vi "Modbus_spy_new.vi"() -> ()   [LabVIEW 2012]
uses:
  Controls/MBA_data.ctl
  <vilib>/Instr/_visa.llb/VISA Configure Serial Port (Instr).vi
panel:
  in  "string":string
  out "MBA data":T1
  in  "Стоп":bool
  out "substring":string
  out "error out":errorcluster
  in  "error in (no error)":errorcluster
  in  "flow control":u16(ring) items=["None"=0, "XON/XOFF"=1, "RTS/CTS"=2, "DTR/DSR"=4]
  in  "stop bits":u16(ring)=20 items=["1.0"=10, "1.5"=15, "2.0"=20]
  in  "parity":u16(ring) items=["None", "Odd", "Even", "Mark", "Space"]
  in  "data bits":u16=8 min=5 max=8 step=1
  in  "VISA resource name":refnum<visa-resource-name>="COM2"
  in  "baud rate":u32=19200
  # "ch1 Т 80л\nch2 нет\nch3 Вытяжка\nch4 Т 30л\nch5 Т 800л\nch6 Охлаждение\nch7 Барботаж\nch8 Т 2000л"
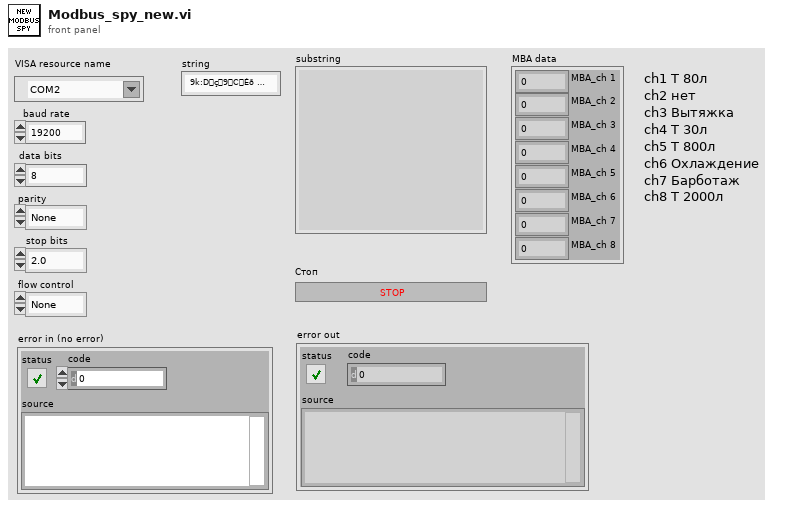
[diagram p1: front panel]
types:
  T1 = typedef "MBA_data.ctl" = cluster{"MBA_ch 1":dbl, "MBA_ch 2":dbl, "MBA_ch 3":dbl, "MBA_ch 4":dbl, "MBA_ch 5":dbl, "MBA_ch 6":dbl, "MBA_ch 7":dbl, "MBA_ch 8":dbl}
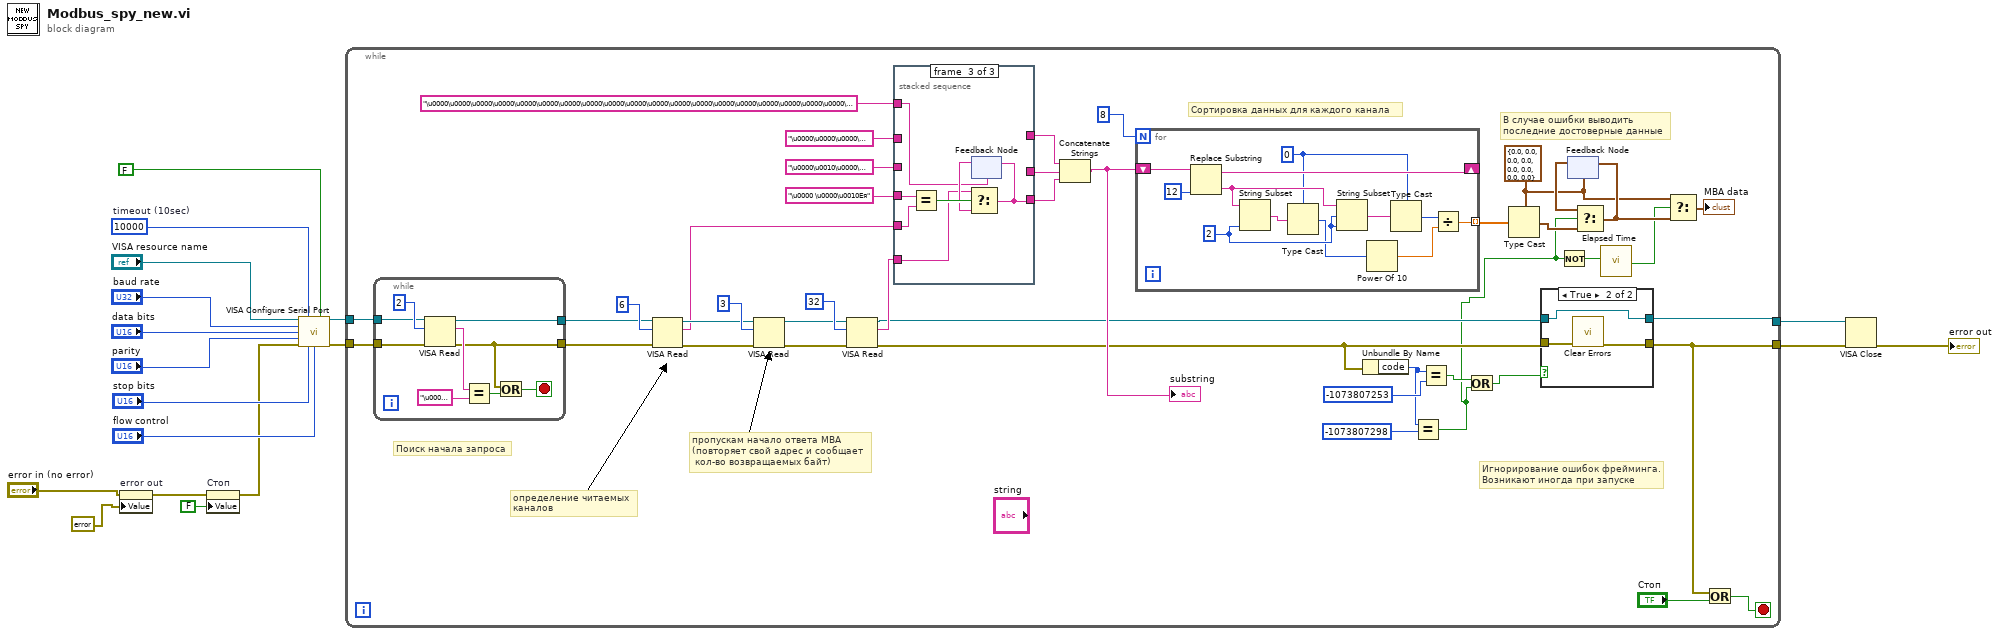
[diagram p0: block diagram]
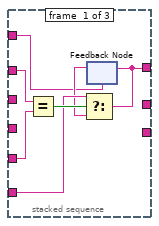
[diagram p3: hidden frame]
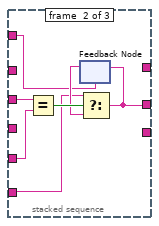
[diagram p4: hidden frame]
diagram:
  w15 = u32 10000  # timeout (10sec)
  n1 = property on="error out" class="Clust (strict)"(error in="error in (no error)", "Value"=errorcluster {"status"=FALSE, "code"=0, "source"=""} ("error in (no error)")) -> (error out=w2:errorcluster)  [unwired: 1 in, 1 out]
  n2 = property on="Стоп" class="Bool (strict)"(error in=w2, "Value"=FALSE ("Стоп")) -> (error out=w5:errorcluster)  [unwired: 1 in, 1 out]
  n3 = call-poly "VISA Configure Serial Port"("VISA resource name"="VISA resource name", "timeout (10sec)"=w15, "Enable Termination\nChar (T)"=FALSE ("Enable Termination\nChar (T)"), "baud rate (9600)"="baud rate", "data bits (8)"="data bits", "parity (0:none)"="parity", "error in (no error)"=w5, "stop bits (10: 1 bit)"="stop bits", "flow control (0:none)"="flow control") -> ("VISA resource name out"=w9:refnum<visa-resource-name>, "error out"=w10:errorcluster)  [unwired: 5 out]
  n4 = while {
    tunnel: w10 -> [w38]
    tunnel: w9 -> [w37]
    tunnel: [w30] -> w8
    tunnel: [w34] -> w7
    stop <- w31 stop-if-true
    w22 = T1 {"MBA_ch 1"=0.0, "MBA_ch 2"=0.0, "MBA_ch 3"=0.0, "MBA_ch 4"=0.0, "MBA_ch 5"=0.0, "MBA_ch 6"=0.0, "MBA_ch 7"=0.0, "MBA_ch 8"=0.0} ("MBA data")
    # "Игнорирование ошибок фрейминга.\nВозникают иногда при запуске"
    # "В случае ошибки выводить \nпоследние достоверные данные"
    # "Сортировка данных для каждого канала"
    # "пропускам начало ответа МВА\n(повторяет свой адрес и сообщает\n кол-во возвращаемых байт)"
    # "определение читаемых \nканалов"
    # "Поиск начала запроса"
    n5 = while {
      tunnel: [w106] -> w59
      tunnel: [w101] -> w58
      tunnel: w38 -> [w100]
      tunnel: w37 -> [w99]
      stop <- w103 stop-if-true
      n6 = VISA Read(VISA resource name=w99, byte count=u32 2, error in (no error)=w100) -> (VISA resource name out=w106:refnum<visa-resource-name>, read buffer=w104:string, error out=w101:errorcluster)  [unwired: 1 out]
      n7 = Equal?(x=w104, y="\u0002\u0003" ("string")) -> (x = y?=w102:bool)
      n8 = Or(x=w101, y=w102) -> (x .or. y?=w103:bool)
    }
    n9 = VISA Read(VISA resource name=w59, byte count=u32 6, error in (no error)=w58) -> (VISA resource name out=w56:refnum<visa-resource-name>, read buffer=w54:string, error out=w55:errorcluster)  [unwired: 1 out]
    n10 = VISA Read(VISA resource name=w56, byte count=u32 3, error in (no error)=w55) -> (VISA resource name out=w51:refnum<visa-resource-name>, error out=w52:errorcluster)  [unwired: 2 out]
    n11 = VISA Read(VISA resource name=w51, byte count=u32 32, error in (no error)=w52) -> (VISA resource name out=w35:refnum<visa-resource-name>, read buffer=w50:string, error out=w33:errorcluster)  [unwired: 1 out]
    n12 = stacked-sequence {
      tunnel: w54 -> [w84 w88 w95]
      tunnel: w50 -> [w81 w89 w96]
      tunnel: "\u0000\u0000\u0000\u0010D5" ("string") -> [w83 _ _]
      tunnel: "\u0000\u0010\u0000\u0010Eр" ("string") -> [_ w87 _]
      tunnel: "\u0000 \u0000\u0010Eя" ("string") -> [_ _ w94]
      tunnel: [w79 _ _] -> w44
      tunnel: [_ w86 _] -> w46
      tunnel: [_ _ w93] -> w45
      tunnel: "\u0000\u0000\u0000\u0000\u0000\u0000\u0000\u0000\u0000\u0000\u0000\u0000\u0000\u0000\u0000\u0000\u0000\u0000\u0000\u0000\u0000\u0000\u0000\u0000\u0000\u0000\u0000\u0000\u0000\u0000\u0000\u0000" ("string") -> [w78 w85 w92]
      frame #0 {
        n13 = Equal?(x=w83, y=w84) -> (x = y?=w82:bool)
        n14 = feedback #1(w78) -> (w80:string)
        n15 = Select(t=w81, s=w82, f=w80) -> (s? t:f=w79:string)
        n16 = feedback-in #1(w79) -> ()
      }
      frame #1 {
        n17 = Equal?(x=w87, y=w88) -> (x = y?=w91:bool)
        n18 = feedback #2(w85) -> (w90:string)
        n19 = Select(t=w89, s=w91, f=w90) -> (s? t:f=w86:string)
        n20 = feedback-in #2(w86) -> ()
      }
      frame #2 {
        n21 = Equal?(x=w94, y=w95) -> (x = y?=w98:bool)
        n22 = feedback #3(w92) -> (w97:string)
        n23 = Select(t=w96, s=w98, f=w97) -> (s? t:f=w93:string)
        n24 = feedback-in #3(w93) -> ()
      }
    }
    n25 = Concatenate Strings(w44, w46, w45) -> (w39:string)
    "substring" <- w39
    n26 = for {
      N: 8 -> [_]
      shift-right: [w75] -> _
      shift-left: w39 -> [w77]
      tunnel: [w66] -> w42 mode=indexing
      w70 = i16 0
      w73 = 2 ("length (rest)")
      n27 = Replace Substring(2:12 ("length (len. of substring)"), 5:w77) -> (0:w72:string, 1:w75:string)  [unwired: 2 in]
      n28 = String Subset(string=w72, length (rest)=w73) -> (substring=w74:string)  [unwired: 1 in]
      n29 = Type Cast(type=w70, x=w74) -> (*(type *) &x=w68:i16)
      n30 = String Subset(string=w72, offset (0)=w73, length (rest)=w73) -> (substring=w71:string)
      n31 = Power Of 10(x=w68) -> (10^x=w67:dbl)
      n32 = Type Cast(type=w70, x=w71) -> (*(type *) &x=w69:i16)
      n33 = Divide(x=w69, y=w67) -> (x/y=w66:dbl)
    }
    n34 = Unbundle By Name(w33) -> ("code"=w28:i32)
    n35 = Equal?(x=w28, y=-1073807298 ("Code")) -> (x = y?=w19:bool)
    n36 = Equal?(x=w28, y=-1073807253) -> (x = y?=w20:bool)
    n37 = Or(x=w20, y=w19) -> (x .or. y?=w26:bool)
    n38 = Type Cast(type=w22, x=w42) -> (*(type *) &x=w41:T1)
    n39 = case shown="True" w26 {
      tunnel: w33 -> [w62 w65]
      tunnel: [w62 w64] -> w30
      tunnel: w35 -> [w61 w63]
      tunnel: [w61 w63] -> w34
      frame False {
      }
      frame True {
        n40 = call <vilib>:"Clear Errors.vi"("error in (no error)"=w65) -> ("error out"=w64:errorcluster)  [unwired: 6 in]
      }
    }
    n41 = Not(x=w19) -> (.not. x?=w25:bool)
    n42 = feedback #4(w22) -> (w40:T1)
    n43 = Select(t=w40, s=w19, f=w41) -> (s? t:f=w24:T1)
    n44 = feedback-in #4(w24) -> ()
    n45 = call "Elapsed Time"("Reset"=w25) -> ("Time has Elapsed"=w21:bool)  [unwired: 11 in, 7 out]
    n46 = Select(t=w22, s=w21, f=w24) -> (s? t:f=→"MBA data":T1)
    n47 = Or(x=w30, y="Стоп") -> (x .or. y?=w31:bool)
  }
  n48 = VISA Close(VISA resource name=w7, error in (no error)=w8) -> (error out=→"error out":errorcluster)
